vi "Device VI 1.1.vi"() -> ()   [LabVIEW 2017]
panel:
  in  "stop":bool
  in  "Number of Samples":i32=500
  in  "Sample Rate":dbl=1000.0
  in  "Stop":bool
  out "Waveform Chart":dynamicdata(graph)
  # "2 Channel Data"
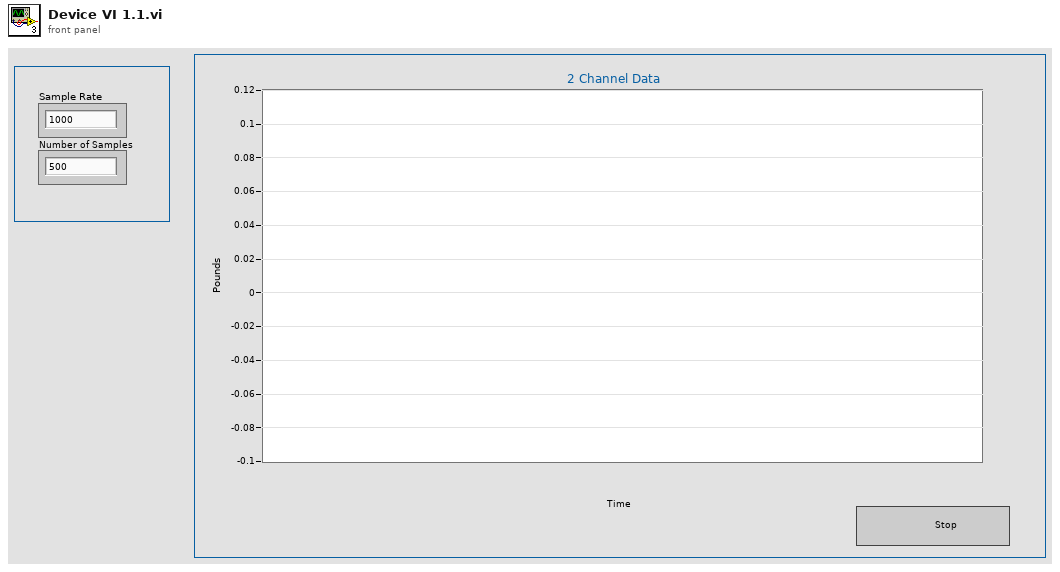
[diagram p1: front panel]
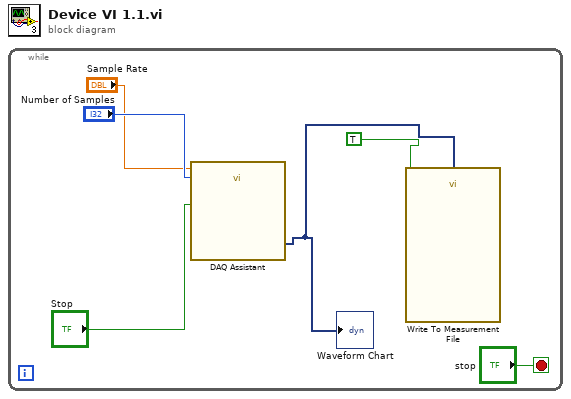
[diagram p0: block diagram]
diagram:
  n1 = while {
    stop <- "stop" stop-if-true
    n2 = call "DAQ Assistant"("rate"="Sample Rate", "number of samples"="Number of Samples", "stop (F)"="Stop") -> ("data"=w1:dynamicdata)  [unwired: 13 in, 3 out]
    "Waveform Chart" <- w1
    n3 = call "Write To Measurement File"("Signals"=w1, "Enable"=TRUE) -> ()  [unwired: 15 in, 3 out]
  }
